vi "base64.vi"(2 "base64 in":string, 3 "string in":string) -> (0 "string out":string, 1 "base64 out":string)   [LabVIEW 2023]
panel:
  # "Man is distinguished, not only by his reason, but by this singular passion from \nother animals, which is a lust of the mind, that by a perseverance of delight in \nthe continued and indefatigable generation of knowledge, exceeds the short v\nehemence of any carnal pleasure."
  # "TWFuIGlzIGRpc3Rpbmd1aXNoZWQsIG5vdCBvbmx5IGJ5IGhpcyByZWFzb24sIGJ1dCBieSB0aGlz\nIHNpbmd1bGFyIHBhc3Npb24gZnJvbSBvdGhlciBhbmltYWxzLCB3aGljaCBpcyBhIGx1c3Qgb2Yg\ndGhlIG1pbmQsIHRoYXQgYnkgYSBwZXJzZXZlcmFuY2Ugb2YgZGVsaWdodCBpbiB0aGUgY29udGlu\ndWVkIGFuZCBpbmRlZmF0aWdhYmxlIGdlbmVyYXRpb24gb2Yga25vd2xlZGdlLCBleGNlZWRzIHRo\nZSBzaG9ydCB2ZWhlbWVuY2Ugb2YgYW55IGNhcm5hbCBwbGVhc3VyZS4="
  # "abc123 => YWJjMTIz"
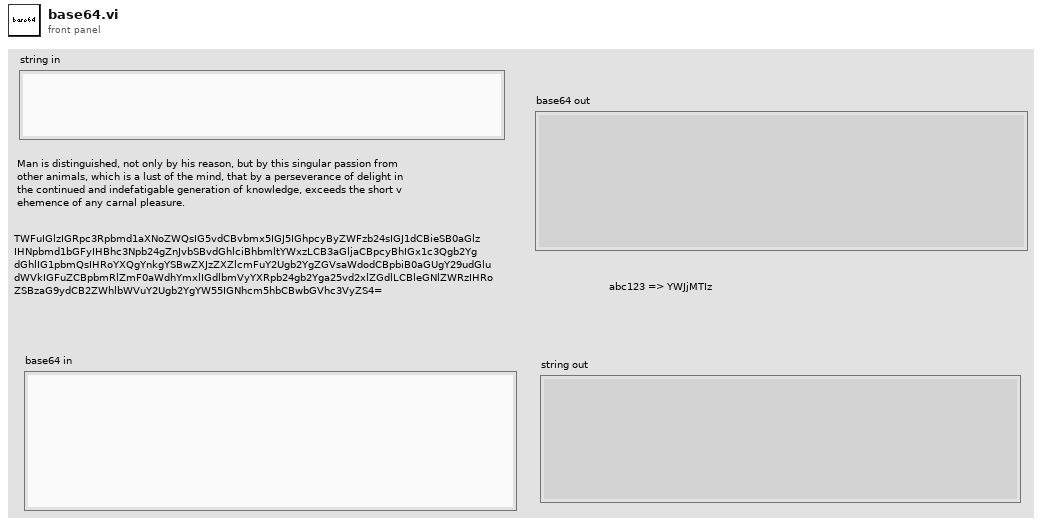
[diagram p1: front panel]
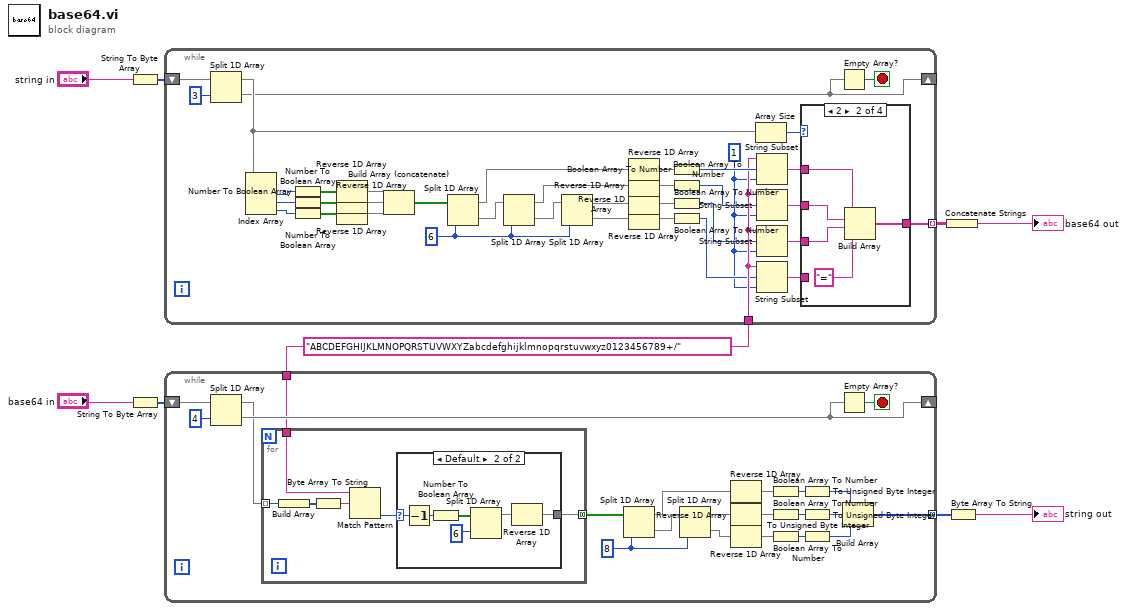
[diagram p0: block diagram]
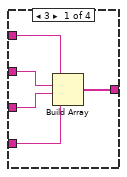
[diagram p3: hidden frame]
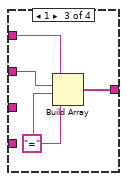
[diagram p4: hidden frame]
diagram:
  w6 = "ABCDEFGHIJKLMNOPQRSTUVWXYZabcdefghijklmnopqrstuvwxyz0123456789+/"
  n1 = String To Byte Array(string="string in") -> (unsigned byte array=w3:u8[])
  n2 = String To Byte Array(string="base64 in") -> (unsigned byte array=w2:u8[])
  n3 = while {
    shift-right: [w10] -> _
    shift-left: w3 -> [w47]
    tunnel: w6 -> [w32]
    tunnel: [w23] -> w4 mode=indexing
    stop <- w46 stop-if-true
    w28 = 1 ("index")
    w40 = 6 ("index")
    n4 = Split 1D Array(array=w47, index=3) -> (first subarray=w21:u8[], second subarray=w10:u8[])
    n5 = Index Array(array=w21) -> (element #1=w43:u8, element #2=w44:u8, element #3=w42:u8)  [unwired: 3 in]
    n6 = Number To Boolean Array(number=w43) -> (Boolean array=w20:bool[])
    n7 = Number To Boolean Array(number=w44) -> (Boolean array=w19:bool[])
    n8 = Number To Boolean Array(number=w42) -> (Boolean array=w18:bool[])
    n9 = Reverse 1D Array(array=w20) -> (reversed array=w17:bool[])
    n10 = Reverse 1D Array(array=w19) -> (reversed array=w16:bool[])
    n11 = Reverse 1D Array(array=w18) -> (reversed array=w15:bool[])
    n12 = Build Array (concatenate)(w17, w16, w15) -> (w41:bool[])
    n13 = Split 1D Array(array=w41, index=w40) -> (first subarray=w37:bool[], second subarray=w39:bool[])
    n14 = Split 1D Array(array=w39, index=w40) -> (first subarray=w36:bool[], second subarray=w38:bool[])
    n15 = Split 1D Array(array=w38, index=w40) -> (first subarray=w35:bool[], second subarray=w34:bool[])
    n16 = Reverse 1D Array(array=w37) -> (reversed array=w14:bool[])
    n17 = Reverse 1D Array(array=w36) -> (reversed array=w13:bool[])
    n18 = Reverse 1D Array(array=w35) -> (reversed array=w12:bool[])
    n19 = Reverse 1D Array(array=w34) -> (reversed array=w11:bool[])
    n20 = Boolean Array To Number(Boolean array=w14) -> (number=w33:u32)
    n21 = Boolean Array To Number(Boolean array=w13) -> (number=w31:u32)
    n22 = Boolean Array To Number(Boolean array=w12) -> (number=w30:u32)
    n23 = Boolean Array To Number(Boolean array=w11) -> (number=w29:u32)
    n24 = Array Size(array=w21) -> (size(s)=w22:i32)
    n25 = String Subset(string=w32, offset (0)=w33, length (rest)=w28) -> (substring=w24:string)
    n26 = String Subset(string=w32, offset (0)=w31, length (rest)=w28) -> (substring=w27:string)
    n27 = String Subset(string=w32, offset (0)=w30, length (rest)=w28) -> (substring=w26:string)
    n28 = String Subset(string=w32, offset (0)=w29, length (rest)=w28) -> (substring=w25:string)
    n29 = case shown="2" w22 {
      tunnel: w27 -> [w52 w57 w61 _]
      tunnel: w26 -> [w51 w56 _ _]
      tunnel: w25 -> [w50 _ _ _]
      tunnel: w24 -> [w49 w55 w60 _]
      tunnel: [w48 w54 w59 _] -> w23
      frame 3 {
        n30 = Build Array(w49, w52, w51, w50) -> (w48:string[])
      }
      frame 2 {
        n31 = Build Array(w55, w57, w56, "=") -> (w54:string[])
      }
      frame 1 {
        w58 = "="
        n32 = Build Array(w60, w61, w58, w58) -> (w59:string[])
      }
      frame Default {
      }
    }
    n33 = Empty Array?(array=w10) -> (empty?=w46:bool)
  }
  n34 = while {
    shift-right: [w80] -> _
    shift-left: w2 -> [w83]
    tunnel: w6 -> [w78]
    tunnel: [w65] -> w1 mode=concatenating
    stop <- w82 stop-if-true
    w76 = 8 ("index")
    n35 = Split 1D Array(array=w83, index=4) -> (first subarray=w79:u8[], second subarray=w80:u8[])
    n36 = for {
      tunnel: w79 -> [w88] mode=indexing
      tunnel: w78 -> [w89]
      tunnel: [w87] -> w75 mode=concatenating
      n37 = Build Array(w88) -> (w86:u8[])
      n38 = Byte Array To String(unsigned byte array=w86) -> (string=w85:string)
      n39 = Match Pattern(string=w89, regular expression=w85) -> (offset past match=w84:i32)  [unwired: 1 in, 3 out]
      n40 = case shown="Default" w84 {
        selector: w84 -> [_ w91]
        tunnel: [_ w95] -> w87
        frame -1 {
        }
        frame Default {
          n41 = Decrement(x=w91) -> (x-1=w90:i32)
          n42 = Number To Boolean Array(number=w90) -> (Boolean array=w94:bool[])
          n43 = Split 1D Array(array=w94, index=6) -> (first subarray=w92:bool[])  [unwired: 1 out]
          n44 = Reverse 1D Array(array=w92) -> (reversed array=w95:bool[])
        }
      }
    }
    n45 = Split 1D Array(array=w75, index=w76) -> (first subarray=w69:bool[], second subarray=w77:bool[])
    n46 = Split 1D Array(array=w77, index=w76) -> (first subarray=w70:bool[], second subarray=w71:bool[])
    n47 = Reverse 1D Array(array=w69) -> (reversed array=w72:bool[])
    n48 = Reverse 1D Array(array=w70) -> (reversed array=w73:bool[])
    n49 = Reverse 1D Array(array=w71) -> (reversed array=w74:bool[])
    n50 = Boolean Array To Number(Boolean array=w72) -> (number=w66:u32)
    n51 = Boolean Array To Number(Boolean array=w73) -> (number=w68:u32)
    n52 = Boolean Array To Number(Boolean array=w74) -> (number=w67:u32)
    n53 = To Unsigned Byte Integer(number=w66) -> (unsigned 8bit integer=w64:u8)
    n54 = To Unsigned Byte Integer(number=w68) -> (unsigned 8bit integer=w63:u8)
    n55 = To Unsigned Byte Integer(number=w67) -> (unsigned 8bit integer=w62:u8)
    n56 = Empty Array?(array=w80) -> (empty?=w82:bool)
    n57 = Build Array(w64, w63, w62) -> (w65:u8[])
  }
  n58 = Concatenate Strings(w4) -> (→"base64 out":string)
  n59 = Byte Array To String(unsigned byte array=w1) -> (string=→"string out":string)
